vi "Write Oscilloscope.vi"(8 "error in (no error)":errorcluster, 10 "Oscilloscope":refnum<class "Oscilloscope.lvclass">, 11 "TopUI in":refnum<class "TopUI.lvclass">) -> (0 "error out":errorcluster, 3 "TopUI out":refnum<class "TopUI.lvclass">)   [LabVIEW 2025, in "TopUI.lvclass"]
uses:
  TopUI.lvclass
  TopUI.lvclass/TopUI.ctl
  Oscilloscope/Oscilloscope.lvclass
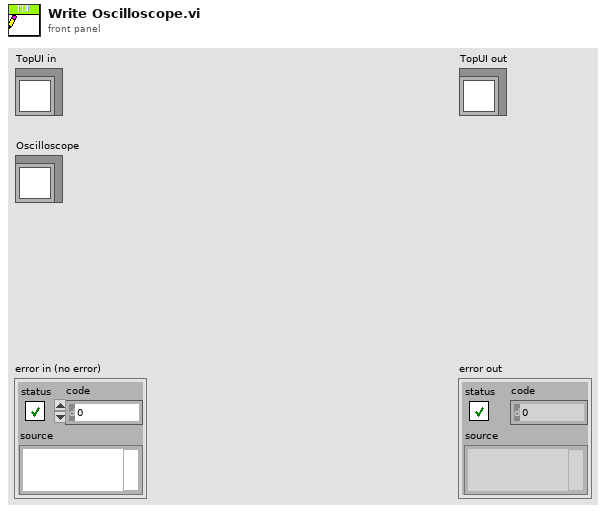
[diagram p1: front panel]
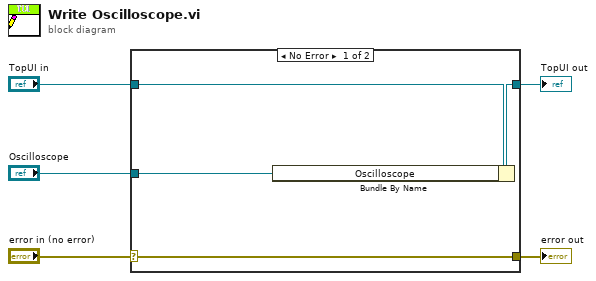
[diagram p0: block diagram]
diagram:
  n1 = case shown="No Error" "error in (no error)" {
    selector: "error in (no error)" -> [w9 w10]
    tunnel: [w9 w10] -> w4
    tunnel: [w7 w11] -> w2
    tunnel: "TopUI in" -> [w8 w11]
    tunnel: "Oscilloscope" -> [w6 _]
    frame No Error {
      n2 = Bundle By Name(cluster=w8, "Oscilloscope"=w6) -> (w7:refnum<class "TopUI.lvclass">)
    }
    frame Error {
    }
  }
  "error out" <- w4
  "TopUI out" <- w2
